vi "TestTemplate.vi"() -> ()   [LabVIEW 2016]
doc: "Contain the test template for creating test cases"
uses:
  <vilib>/SLL Drona/APIs/Stimulus/ControlValue/SetValueAuto.vi
  <vilib>/SLL Drona/APIs/Assert/AssertControlValue/Equal.vi
  <vilib>/SLL Drona/Drona.lvlib
  <vilib>/addons/_JKI Toolkits/Caraya/classes/Test/Test.lvclass
  <vilib>/SLL Drona/APIs/Stimulus/ControlValue/ControlValue.lvlib
  <vilib>/SLL Drona/APIs/Assert/AssertControlValue/AssertControlValue.lvlib
panel:
  out "error out":errorcluster
  in  "error in (no error)":errorcluster
  # "Test Template"
  # "Note:  All the testcase names should start \nwith prefix \"Test\""
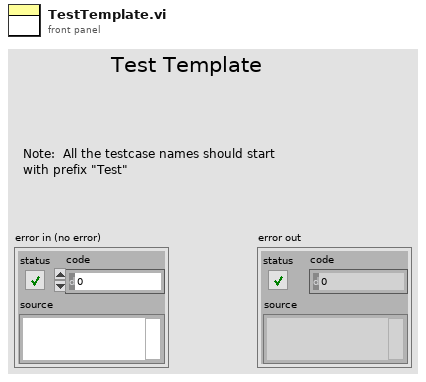
[diagram p1: front panel]
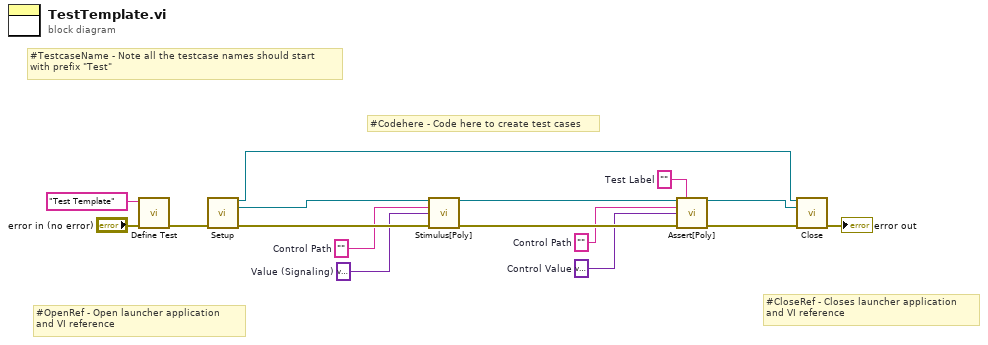
[diagram p0: block diagram]
diagram:
  w2 = ""  # Test Label
  w3 = variant  # Control Value
  w4 = ""  # Control Path
  w5 = variant  # Value (Signaling)
  w6 = ""  # Control Path
  # "#CloseRef - Closes launcher application\nand VI reference"
  # "#OpenRef - Open launcher application\nand VI reference"
  # "#Codehere - Code here to create test cases"
  # "#TestcaseName - Note all the testcase names should start \nwith prefix \"Test\""
  n1 = call <vilib>:"Define Test.vi"("error in (no error)"="error in (no error)", "Label (VI Title)"="Test Template") -> ("error out"=w16:errorcluster)  [unwired: 9 in]
  n2 = call <vilib>:"Setup.vi"("error in"=w16) -> ("Application Ref"=w10:refnum<vi>, "VI Reference Out"=w9:refnum<vi>, "error out"=w15:errorcluster)  [unwired: 12 in]
  n3 = call-poly <vilib>:"Stimulus[Poly].vi"("VI Reference In"=w9, "Control Path"=w6, "Value (Signaling)"=w5, "error in"=w15) -> ("VI Reference Out"=w8:refnum<vi>, "error out"=w14:errorcluster)  [unwired: 10 in]
  n4 = call-poly <vilib>:"Assert[Poly].vi"("VI Reference In"=w8, "Test Label"=w2, "Control Path"=w4, "Control Value"=w3, "Error In"=w14) -> ("VI Reference Out"=w7:refnum<vi>, "Error Out"=w13:errorcluster)  [unwired: 9 in]
  n5 = call <vilib>:"Close.vi"("Application Ref"=w10, "VI Reference"=w7, "error in"=w13) -> ("error out"=→"error out":errorcluster)  [unwired: 12 in]
